vi "MM6.FormatScanStep.vi"(1 "Name":string, 3 "Value":dbl, 4 "FctName":string, 5 "SetSpecial":string) -> (15 "SetSpecial":string, 17 "byteArray out":T1)   [LabVIEW 2014, in "MM6.lvlib"]
uses:
  MM6.lvlib
  CSCore/CSSystem/CoreDefs/CoreDefs.rawDataType.ctl
  CSCore/CSSystem/CoreLib/CoreLib.double 2 byte array.vi
  CSCore/CSSystem/CoreLib/CoreLib.string 2 byte array.vi
  CSCore/CSSystem/CoreLib/CoreLib.int 2 byte array.vi
  CSCore/CSSystem/CoreLib/CoreLib.short 2 byte array.vi
  CSCore/CSSystem/CoreLib/CoreLib.lvlib
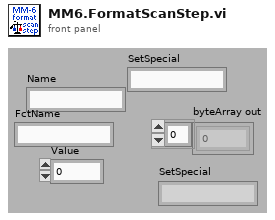
[diagram p1: front panel]
types:
  T1 = typedef "CoreDefs.rawDataType.ctl" = i8[]
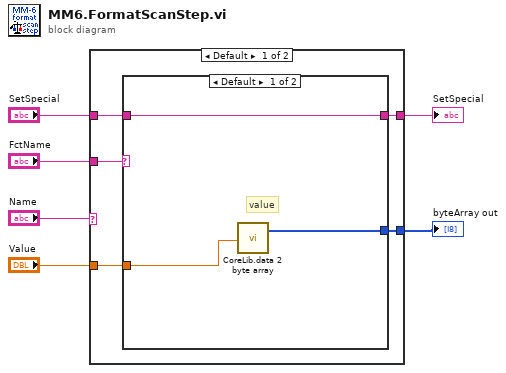
[diagram p0: block diagram]
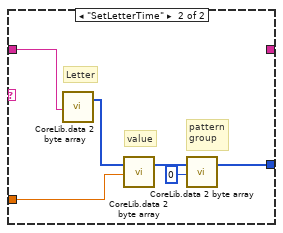
[diagram p2: hidden frame]
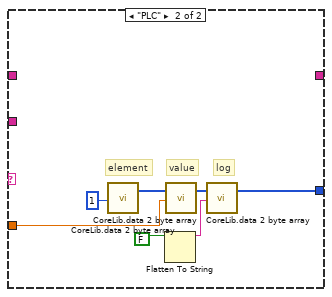
[diagram p3: hidden frame]
diagram:
  n1 = case shown="Default" "Name" {
    tunnel: "Value" -> [w10 w22]
    tunnel: [w11 w25] -> w4
    tunnel: "FctName" -> [w9 _]
    tunnel: "SetSpecial" -> [w8 _]
    tunnel: [w7 _] -> w1
    frame Default {
      n2 = case shown="Default" w9 {
        tunnel: [w14 w17] -> w11
        tunnel: w10 -> [w13 w20]
        tunnel: w8 -> [w12 w15]
        tunnel: [w12 _] -> w7
        frame Default {
          # "value"
          n3 = call-poly "CoreLib.data 2 byte array.vi"("f64"=w13) -> ("byteArray out"=w14:T1)  [unwired: 18 in]
        }
        frame "SetLetterTime" {
          # "Letter"
          # "pattern\ngroup"
          # "value"
          n4 = call-poly "CoreLib.data 2 byte array.vi"("string"=w15) -> ("byteArray out"=w19:T1)  [unwired: 18 in]
          n5 = call-poly "CoreLib.data 2 byte array.vi"("byteArray"=w19, "f64"=w20) -> ("byteArray out"=w18:T1)  [unwired: 17 in]
          n6 = call-poly "CoreLib.data 2 byte array.vi"("byteArray"=w18, "i32"=0) -> ("byteArray out"=w17:T1)  [unwired: 17 in]
        }
      }
    }
    frame "PLC" {
      # "log"
      # "value"
      # "element"
      n7 = call-poly "CoreLib.data 2 byte array.vi"("i16"=i16 1) -> ("byteArray out"=w24:T1)  [unwired: 18 in]
      n8 = Flatten To String(anything=FALSE) -> (data string=w21:string)  [unwired: 3 in, 2 out]
      n9 = call-poly "CoreLib.data 2 byte array.vi"("byteArray"=w24, "f64"=w22) -> ("byteArray out"=w26:T1)  [unwired: 17 in]
      n10 = call-poly "CoreLib.data 2 byte array.vi"("byteArray"=w26, "string"=w21) -> ("byteArray out"=w25:T1)  [unwired: 17 in]
    }
  }
  "byteArray out" <- w4
  "SetSpecial" <- w1
